vi "Init Acquisition.vi"(0 "Lens Mode":string="Transmission", 2 "element_set":string, 5 "Pass Energy":dbl=150.0, 7 "Region":T1={"fixed_"=0, "highEnergy_"=500.0, "lowEnergy_"=0.0, "centerEnergy_"=0.0, "energyStep_"=10.0, "dwellTime_"=67}, 9 "Detector Region":T2={"firstXChannel_"=1, "lastXChannel_"=1392, "firstYChannel_"=1, "lastYChannel_"=519, "slices_"=519, "adcMode_"=1}, 11 "error in (no error)":errorcluster) -> (3 "element_set out":string, 4 "Lens Mode out":string="Transmission", 6 "Pass Energy out":dbl=150.0, 8 "Region out":T1={"fixed_"=0, "highEnergy_"=500.0, "lowEnergy_"=0.0, "centerEnergy_"=0.0, "energyStep_"=10.0, "dwellTime_"=67}, 10 "Detector Region out":T2={"firstXChannel_"=1, "lastXChannel_"=1392, "firstYChannel_"=1, "lastYChannel_"=519, "slices_"=519, "adcMode_"=1}, 15 "error out":errorcluster)   [LabVIEW 2018]
uses:
  SesWrapper/SesWrapper.lvlib
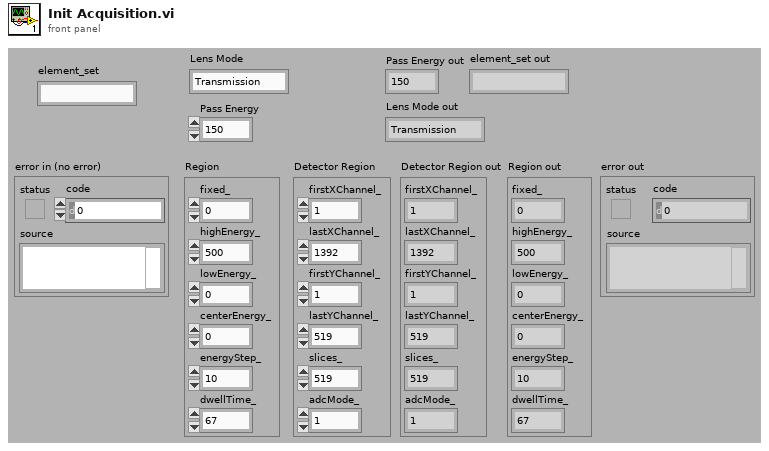
[diagram p1: front panel]
types:
  T1 = cluster{"fixed_":u8, "highEnergy_":dbl, "lowEnergy_":dbl, "centerEnergy_":dbl, "energyStep_":dbl, "dwellTime_":i32}
  T2 = cluster{"firstXChannel_":i32, "lastXChannel_":i32, "firstYChannel_":i32, "lastYChannel_":i32, "slices_":i32, "adcMode_":u8}
  T3 = cluster{"fixed_":u8, "@dummy control@":i8, "@dummy control@":i8, "@dummy control@":i8, "@dummy control@":i8, "@dummy control@":i8, "@dummy control@":i8, "@dummy control@":i8, "highEnergy_":dbl, "lowEnergy_":dbl, "centerEnergy_":dbl, "energyStep_":dbl, "dwellTime_":i32}
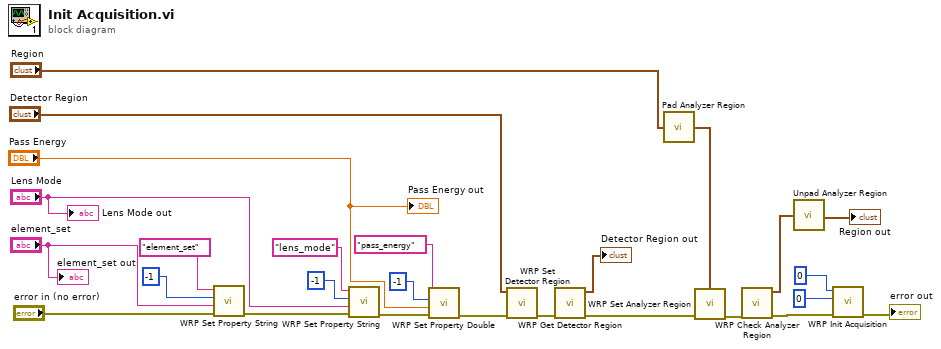
[diagram p0: block diagram]
diagram:
  n1 = call "WRP Set Property String.vi"("error in (no error)"="error in (no error)", "value"="element_set", "index"=-1, "property"="element_set") -> ("error out"=w4:errorcluster)  [unwired: 6 in, 1 out]
  n2 = call "WRP Set Property String.vi"("error in (no error)"=w4, "value"="Lens Mode", "index"=-1, "property"="lens_mode") -> ("error out"=w22:errorcluster)  [unwired: 6 in, 1 out]
  n3 = call "WRP Set Property Double.vi"("error in (no error)"=w22, "value"="Pass Energy", "index"=-1, "property"="pass_energy") -> ("error out"=w21:errorcluster)  [unwired: 6 in, 1 out]
  n4 = call "WRP Set Detector Region.vi"("error in (no error)"=w21, "detectorRegion"="Detector Region") -> ("error out"=w14:errorcluster)  [unwired: 8 in, 1 out]
  n5 = call "WRP Get Detector Region.vi"("error in (no error)"=w14) -> ("error out"=w13:errorcluster, "value"=→"Detector Region out":T2)  [unwired: 8 in, 1 out]
  n6 = call "Pad Analyzer Region.vi"("Analyzer Region"="Region") -> ("Analyzer Region out"=w15:T3)  [unwired: 4 in]
  n7 = call "WRP Set Analyzer Region.vi"("error in (no error)"=w13, "analyzerRegion"=w15) -> ("error out"=w11:errorcluster)  [unwired: 8 in, 1 out]
  n8 = call "WRP Check Analyzer Region.vi"("error in (no error)"=w11) -> ("error out"=w10:errorcluster, "analyzerRegion"=w6:T3)  [unwired: 5 in, 4 out]
  n9 = call "Unpad Analyzer Region.vi"("Analyzer Region"=w6) -> ("Analyzer Region out"=→"Region out":T1)  [unwired: 4 in]
  n10 = call "WRP Init Acquisition.vi"("error in (no error)"=w10, "block_RegionReady"=u8 0 ("block_PointReady"), "block_PointReady"=u8 0 ("block_RegionReady")) -> ("error out"=→"error out":errorcluster)  [unwired: 7 in, 1 out]
  "Pass Energy out" <- "Pass Energy"
  "Lens Mode out" <- "Lens Mode"
  "element_set out" <- "element_set"
